vi "Scan DQMH Modules and create Maps.vi"(8 "error in":errorcluster, 11 "Project":refnum<vi>) -> (0 "error out":errorcluster, 1 "Tree Map out":T1, 2 "map ref out":map{string, refnum<vi>}(c390), 3 "DQMH Modules Info":T2, 4 "Cancelled?":bool)   [LabVIEW 2020, in "Panther Dashboard.lvlib"]
doc: "Gets the Singleton and Cloneable references and creates a list of each type of DQMH Modules"
uses:
  Panther Dashboard.lvlib
  DQMH Modules Info--cluster.ctl
  Module type--enum.ctl
  <vilib>/National Instruments/Tree Map/Tree Map Data.ctl
  Event types--enum.ctl
  <vilib>/National Instruments/Tree Map/Tree Map.lvlib
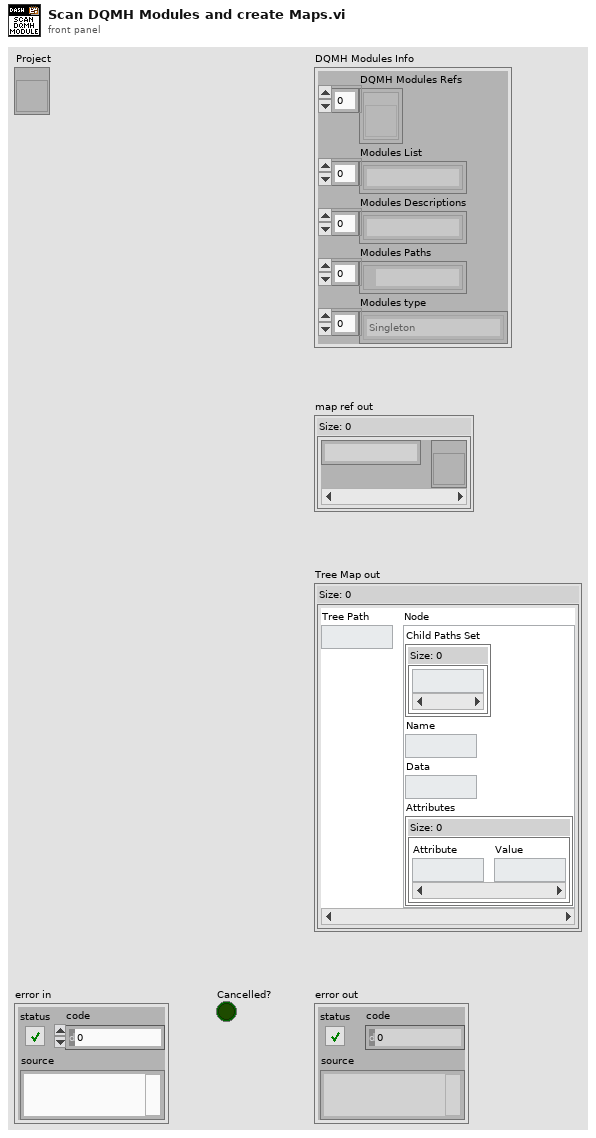
[diagram p1: front panel]
types:
  T1 = typedef "Tree Map.lvlib/Tree Map Data.ctl" = map{string, cluster{"Child Paths Set":set{string}, "Name":string, "Data":string, "Attributes":map{string, string}}}
  T2 = typedef "Panther Dashboard.lvlib/DQMH Modules Info--cluster.ctl" = cluster{"DQMH Modules Refs":refnum<vi>[], "Modules List":string[], "Modules Descriptions":string[], "Modules Paths":path[], "Modules type":T3[]}
  T3 = typedef "Panther Dashboard.lvlib/Module type--enum.ctl" = enum16{"Singleton", "Cloneable"}
  T4 = typedef "Panther Dashboard.lvlib/Event types--enum.ctl" = enum16{"Request", "Request and Wait for Reply", "Broadcast"}
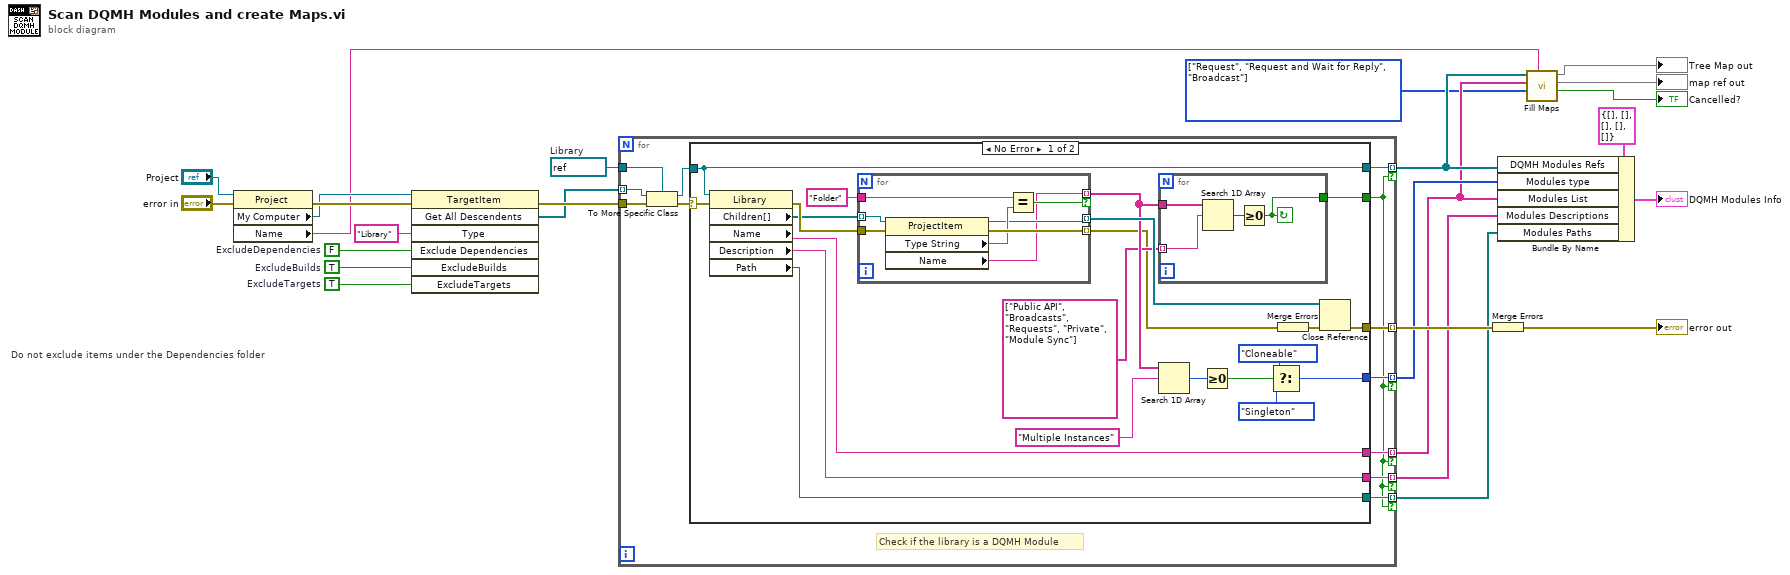
[diagram p0: block diagram]
diagram:
  w6 = T4[] [enum."Request", enum."Request and Wait for Reply", enum."Broadcast"] items=["Request", "Request and Wait for Reply", "Broadcast"] ("Event Types")
  w17 = refnum<vi> refnum  # Library
  w18 = FALSE  # ExcludeDependencies
  w19 = TRUE  # ExcludeTargets
  w20 = TRUE  # ExcludeBuilds
  # "Do not exclude items under the Dependencies folder"
  n1 = property class="Project"(reference="Project", error in="error in") -> (error out=w24:errorcluster, "My Computer"=w21:refnum<vi>, "Name"=w1:string)  [unwired: 1 out]
  n2 = invoke class="TargetItem" method="Get All Descendents"(reference=w21, error in=w24, "Type"="Library", "Exclude Dependencies"=w18, "ExcludeBuilds"=w20, "ExcludeTargets"=w19) -> (error out=w25:errorcluster, "All Descendents"=w16:refnum<vi>[])  [unwired: 1 in, 5 out]
  n3 = for {
    tunnel: w17 -> [w34]
    tunnel: [w33] -> w8 mode=indexing if=w26
    tunnel: w16 -> [w31] mode=indexing
    tunnel: [w36] -> w15 mode=indexing
    tunnel: w25 -> [w35]
    tunnel: [w30] -> w12 mode=indexing if=w26
    tunnel: [w29] -> w7 mode=indexing if=w26
    tunnel: [w28] -> w11 mode=indexing if=w26
    tunnel: [w27] -> w10 mode=indexing if=w26
    # "Check if the library is a DQMH Module"
    n4 = To More Specific Class(target class=w34, reference=w31, error in=w35) -> (specific class reference=w32:refnum<vi>, error out=w37:errorcluster)
    n5 = case shown="No Error" w37 {
      selector: w37 -> [w58 _]
      tunnel: w32 -> [w45 _]
      tunnel: [w54 _] -> w26
      tunnel: [w45 _] -> w33
      tunnel: [w57 _] -> w36
      tunnel: [w39 _] -> w30
      tunnel: [w44 _] -> w29
      tunnel: [w43 _] -> w28
      tunnel: [w42 _] -> w27
      frame No Error {
        n6 = property class="Library"(reference=w45, error in=w58) -> (error out=w56:errorcluster, "Children[]"=w52:refnum<vi>[], "Name"=w44:string, "Description"=w43:string, "Path"=w42:path)  [unwired: 1 out]
        n7 = for {
          tunnel: [w63] -> w48 mode=indexing if=w64
          tunnel: w56 -> [w70]
          tunnel: [w69] -> w46 mode=indexing
          tunnel: [w66] -> w51 mode=indexing
          tunnel: w52 -> [w68] mode=indexing
          tunnel: "Folder" ("Type") -> [w65]
          n8 = property class="ProjectItem"(reference=w68, error in=w70) -> (reference out=w66:refnum<vi>, error out=w69:errorcluster, "Type String"=w67:string, "Name"=w63:string)
          n9 = Equal?(x=w65, y=w67) -> (x = y?=w64:bool)
        }
        n10 = for {
          tunnel: string[] ["Public API", "Broadcasts", "Requests", "Private", "Module Sync"] -> [w62] mode=indexing
          tunnel: w48 -> [w61]
          tunnel: [w59] -> w54
          stop <- w59 continue-if-true
          n11 = Search 1D Array(1D array=w61, element=w62) -> (index of element=w60:i32)  [unwired: 1 in]
          n12 = Greater Or Equal To 0?(x=w60) -> (x >= 0?=w59:bool)
        }
        n13 = Search 1D Array(1D array=w48, element="Multiple Instances") -> (index of element=w50:i32)  [unwired: 1 in]
        n14 = Greater Or Equal To 0?(x=w50) -> (x >= 0?=w41:bool)
        n15 = Select(t=Module_type--enum."Cloneable", s=w41, f=Module_type--enum."Singleton" ("Module type")) -> (s? t:f=w39:T3)
        n16 = Merge Errors(w46) -> (w55:errorcluster)
        n17 = Close Reference(reference=w51, error in (no error)=w55) -> (error out=w57:errorcluster)
      }
      frame Error {
      }
    }
  }
  n18 = Merge Errors(w15) -> (→"error out":errorcluster)
  n19 = Bundle By Name(cluster=T2 {"DQMH Modules Refs"=[], "Modules List"=[], "Modules Descriptions"=[], "Modules Paths"=[], "Modules type"=[]} ("DQMH Modules Info"), "DQMH Modules Refs"=w8, "Modules type"=w12, "Modules List"=w7, "Modules Descriptions"=w11, "Modules Paths"=w10) -> (→"DQMH Modules Info":T2)
  n20 = call "Fill Maps.vi"("Project Selected"=w1, "Event Types"=w6, "Module names"=w7, "DQMH Modules"=w8) -> ("Cancelled?"=→"Cancelled?":bool, "map ref out"=→"map ref out":map{string, refnum<vi>}, "Tree Map out"=→"Tree Map out":T1)  [unwired: 5 in]
